vi "Read_Camera.vi"(0 "error in":errorcluster, 2 "Camera":T3, 3 "node":string) -> (1 "error out":errorcluster, 4 "image data":T1)   [LabVIEW 2012]
doc: "Get an image from one of Baxter's hand cameras. \n\nIt is highly recommended that you are connected to baxter via ethernet rather than over wireless when doing this."
uses:
  <userlib>/rosforlv/ROS/Code/SubVIs/BaxterCamera.ctl
  <vilib>/picture/picture.llb/imagedata.ctl
  <userlib>/rosforlv/ROS/Code/Console/Servers/ServerSubs/TopicDef.ctl
  <userlib>/rosforlv/ROS/Code/SubVIs/_ROSDirection.ctl
panel:
  out "ROS Image":T2
  out "image":picture
  out "Reply":string
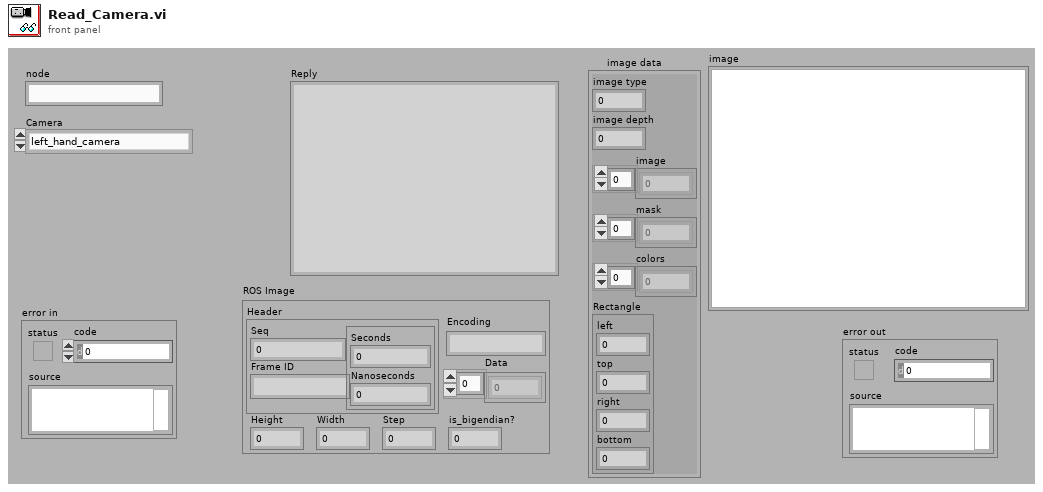
[diagram p1: front panel]
types:
  T1 = typedef "imagedata.ctl" = cluster{"image type":i32, "image depth":i32, "image":u8[], "mask":u8[], "colors":u32[], "Rectangle":cluster{"left":i16, "top":i16, "right":i16, "bottom":i16}}
  T2 = cluster{"Header":cluster{"Seq":u32, "Frame ID":string, cluster{"Seconds":i32, "Nanoseconds":i32}}, "Height":u32, "Width":u32, "is_bigendian?":u8, "Step":u32, "Data":u8[], "Encoding":string}
  T3 = typedef "BaxterCamera.ctl" = enum16{"left_hand_camera", "right_hand_camera", "head_camera"}
  T4 = typedef "TopicDef.ctl" = cluster{"Topic":string, "Type":string, "Action":T5, "Update (ms)":u16, "write queue":u16}
  T5 = typedef "_ROSDirection.ctl" = enum16{"Node", "Publisher", "Subscriber", "Service Client"}
  T6 = typedef "_ROSControl.ctl" = cluster{"topic port":u16, "Node":string, "topic":string, "type":string, "node port":u32, "error ":errorcluster, "Direction":T5, "APIs":string[], "Update (ms)":u16, "write queue":u16}
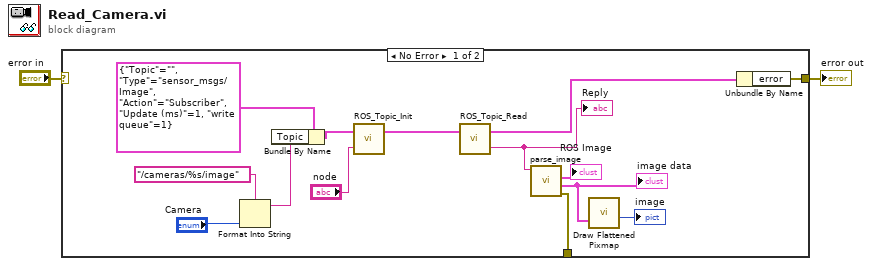
[diagram p0: block diagram]
diagram:
  n1 = case shown="No Error" "error in" {
    selector: "error in" -> [_ w17]
    tunnel: [w16 w17] -> w2
    tunnel: [w10 _] -> _
    frame No Error {
      n2 = Format Into String(format string="/cameras/%s/image" ("topic"), "Camera") -> (resulting string=w7:string)  [unwired: 2 in, 1 out]
      n3 = Bundle By Name(cluster=T4 {"Topic"="", "Type"="sensor_msgs/Image", "Action"=enum."Subscriber", "Update (ms)"=1, "write queue"=1} ("Definitions"), "Topic"=w7) -> (w6:T4)
      n4 = call <userlib>:"ROS_Topic_Init.vi"("node"="node", "Definitions"=w6) -> ("ROS out"=w14:T6)  [unwired: 1 in]
      n5 = call <userlib>:"ROS_Topic_Read.vi"("ROS in"=w14) -> ("Reply"=w11:string, "ROS out"=w13:T6)  [unwired: 1 in]
      "Reply" <- w11
      n6 = call <userlib>:"parse_image.vi"("msg in"=w11) -> ("error out"=w10:errorcluster, "image data"=w3:T1, "ROS Image"=→"ROS Image":T2)  [unwired: 3 in, 1 out]
      "image data" <- w3
      n7 = call <vilib>:"Draw Flattened Pixmap.vi"("image data"=w3) -> ("new picture"=→"image":picture)  [unwired: 8 in]
      n8 = Unbundle By Name(w13) -> ("error"=w16:errorcluster)
    }
    frame Error {
    }
  }
  "error out" <- w2
